vi "testLogMsg.vi"(8 "error in (no error)":errorcluster) -> (0 "error out":errorcluster)   [LabVIEW 2018]
uses:
  src/Logger/Logger.lvclass
  <vilib>/addons/_JKI Toolkits/Caraya/classes/Assert/Assert Equal Value_Variant.vi
  <vilib>/addons/_JKI Toolkits/Caraya/classes/Test/Test.lvclass
  <vilib>/addons/_JKI Toolkits/Caraya/classes/Assert/Assert.lvclass
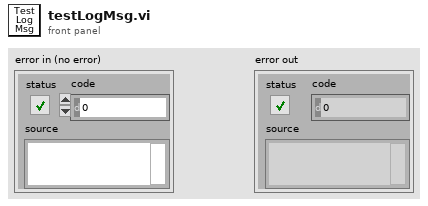
[diagram p1: front panel]
types:
  T1 = enum16{"NOTSET", "DEBUG", "INFO", "WARNING", "ERROR", "CRITICAL"}
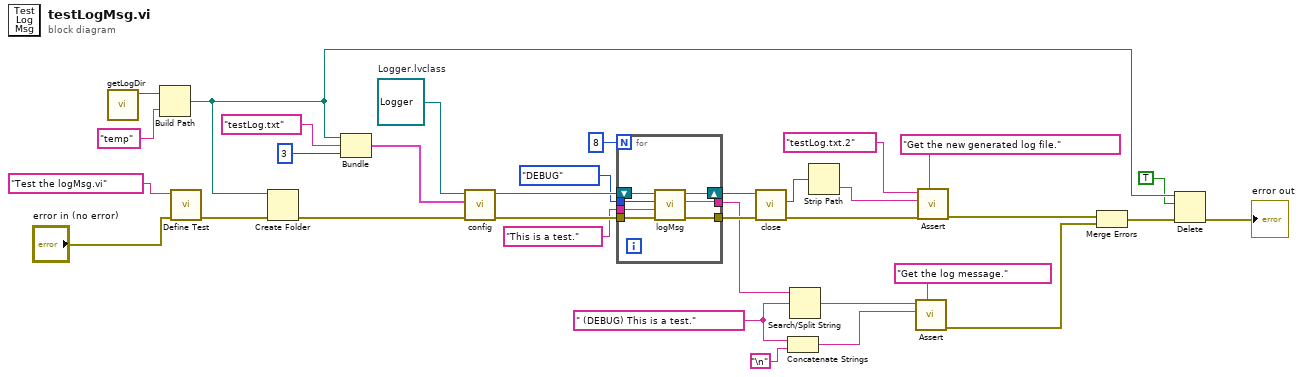
[diagram p0: block diagram]
diagram:
  w11 = " (DEBUG) This is a test."
  w32 = refnum<class "Logger.lvclass"> refnum  # Logger.lvclass
  n1 = call "getLogDir.vi"() -> ("dirLog"=w8:path)  [unwired: 11 in]
  n2 = Build Path(base path=w8, name or relative path="temp") -> (appended path=w2:path)
  n3 = call <vilib>:"Define Test.vi"("error in (no error)"="error in (no error)", "Label (VI Title)"="Test the logMsg.vi") -> ("error out"=w6:errorcluster)  [unwired: 9 in]
  n4 = Create Folder(path (use dialog)=w2, error in=w6) -> (error out=w5:errorcluster)  [unwired: 1 in, 2 out]
  n5 = Bundle("appended path"=w2, "testLog.txt", 3) -> (w29:cluster{"appended path":path, string, i32})  [unwired: 1 in]
  n6 = call "config.vi"("error in (no error)"=w5, "confData"=w29, "Logger in"=w32) -> ("error out"=w28:errorcluster, "Logger out"=w27:refnum<class "Logger.lvclass">)  [unwired: 7 in]
  n7 = for {
    N: 8 -> [_]
    tunnel: w28 -> [w40]
    tunnel: T1."DEBUG" ("type") -> [w39]
    tunnel: "This is a test." -> [w38]
    tunnel: [w36] -> w22
    tunnel: [w35] -> w16
    shift-right: [w37] -> w23
    shift-left: w27 -> [w41]
    n8 = call "logMsg.vi"("error in (no error)"=w40, "msg"=w38, "type"=w39, "Logger in"=w41) -> ("error out"=w36:errorcluster, "msgLog"=w35:string, "Logger out"=w37:refnum<class "Logger.lvclass">)  [unwired: 5 in]
  }
  n9 = call "close.vi"("error in (no error)"=w22, "Logger in"=w23) -> ("error out"=w21:errorcluster, "filePathClosed"=w20:path)  [unwired: 7 in, 1 out]
  n10 = Concatenate Strings(w11, "\n") -> (w9:string)
  n11 = Search/Split String(string=w16, search string/char (-)=w11) -> (match + rest of string=w10:string)  [unwired: 1 in, 2 out]
  n12 = Strip Path(path=w20) -> (name=w19:string)  [unwired: 1 out]
  n13 = call-poly <vilib>:"Assert.vi"("Label"="Get the log message.", "Y"=w9, "X"=w10) -> ("error out"=w13:errorcluster)  [unwired: 8 in]
  n14 = call-poly <vilib>:"Assert.vi"("Label"="Get the new generated log file.", "error in (no error)"=w21, "Y"=w19, "X"="testLog.txt.2") -> ("error out"=w14:errorcluster)  [unwired: 7 in]
  n15 = Merge Errors(w14, w13) -> (w4:errorcluster)
  n16 = Delete(path (use dialog)=w2, entire hierarchy (F)=TRUE, error in=w4) -> (error out=→"error out":errorcluster)  [unwired: 2 in, 2 out]
